vi "Write Report.vi"(8 "error in (no error)":errorcluster, 10 "Resource In":variant, 11 "Analyze Results Total Counts in":refnum<class "Analyze Results Total Counts.lvclass">) -> (0 "error out":errorcluster, 2 "Resource Out":variant, 3 "Analyze Results Total Counts out":refnum<class "Analyze Results Total Counts.lvclass">)   [LabVIEW 2014, in "Analyze Results Total Counts.lvclass"]
uses:
  Analyze Results Total Counts.lvclass
  Results Base/Analyze Results Base.lvclass
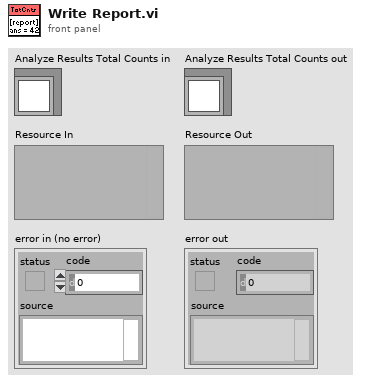
[diagram p1: front panel]
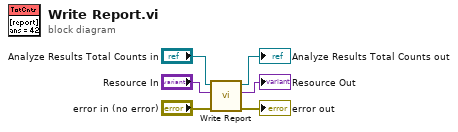
[diagram p0: block diagram]
diagram:
  n1 = call-parent "Write Report.vi"("error in (no error)"="error in (no error)", "Resource In"="Resource In", "Analyze Results Base in"="Analyze Results Total Counts in") -> ("error out"=→"error out":errorcluster, "Resource Out"=→"Resource Out":variant, "Analyze Results Base out"=→"Analyze Results Total Counts out":refnum<class "Analyze Results Total Counts.lvclass">)  [unwired: 6 in]
